vi "DangerousEnemyCriteria.vi"(8 "error in (no error)":errorcluster, 10 "Point":dbl[](array[numeric]), 11 "TestObjetive in":refnum<class "TestObjetive.lvclass">) -> (0 "error out":errorcluster, 2 "evaluation":dbl, 3 "TestObjetive out":refnum<class "TestObjetive.lvclass">)   [LabVIEW 2023, in "TestObjetive.lvclass"]
uses:
  TestObjetive.lvclass
  TestObjetive.lvclass/TestObjetive.ctl
  Game_class/Game.lvclass/Game.ctl
  Object_class/Object.lvclass/Object.ctl
  Team_class/Team.lvclass/Team.ctl
  Object_class/Read x.vi
  Object_class/Read y.vi
  Game_class/Read BallRef.vi
  Game_class/Read EnemyRef.vi
  Team_class/Read RobotRef.vi
  Object_class/Read position(x,y).vi
  Enemy_class/Enemy.lvclass
  C:/Users/ebert/Documents/codes/SSL/repo/SSL_AI/Team_class/Team.lvclass
  Ball_class/Ball.lvclass
  C:/Users/ebert/Documents/codes/SSL/repo/SSL_AI/Object_class/Object.lvclass
  Robot_class/Robot.lvclass
  Utilities_class/Utilities.lvclass
  Game_class/Game.lvclass
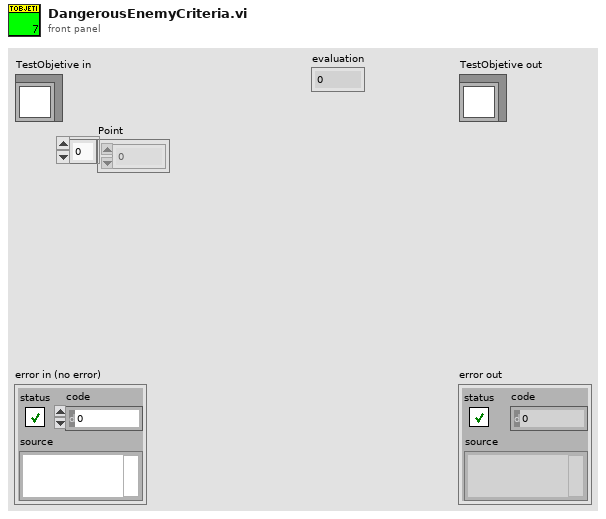
[diagram p1: front panel]
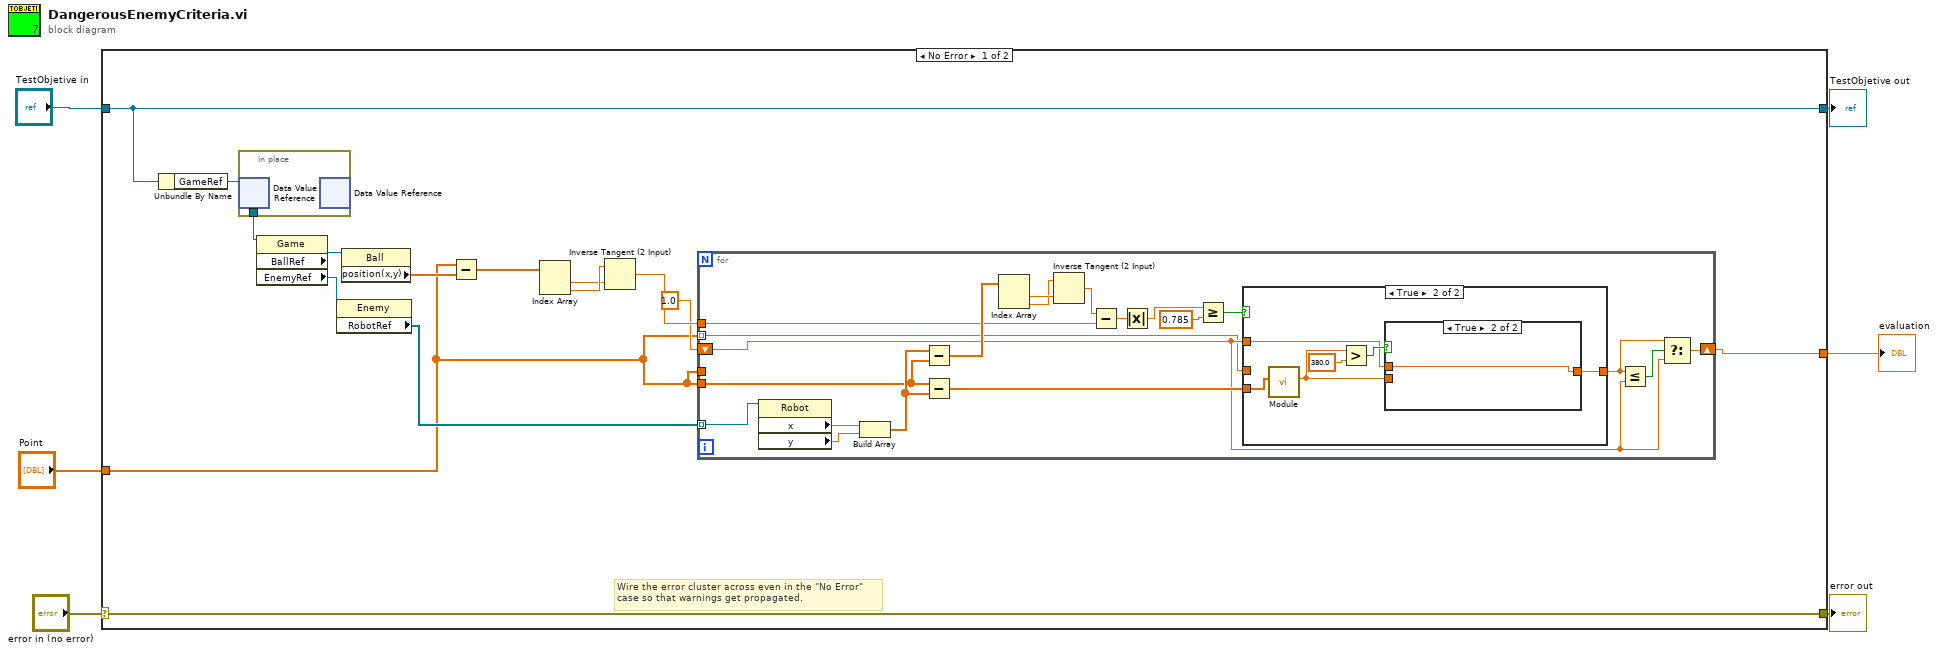
[diagram p0: block diagram]
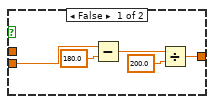
[diagram p3: hidden frame]
diagram:
  n1 = case shown="No Error" "error in (no error)" {
    selector: "error in (no error)" -> [w21 w57]
    tunnel: [w21 w57] -> w5
    tunnel: [w15 w56] -> w3
    tunnel: "TestObjetive in" -> [w15 w56]
    tunnel: "Point" -> [w8 _]
    tunnel: [w7 _] -> w1
    frame No Error {
      # "Wire the error cluster across even in the \"No Error\"\ncase so that warnings get propagated."
      n2 = Unbundle By Name(w15) -> ("GameRef"=w14:refnum<data-value>)
      n3 = in-place {
        in-place-border: [w22] -> w13
        n4 = in-place-dvr #1(w14) -> (w22:refnum<class "Game.lvclass">)  [unwired: 1 out]
        n5 = in-place-dvr #1() -> ()  [unwired: 1 in, 2 out]
      }
      n6 = property class="Game"(reference=w13) -> ("BallRef"=w12:refnum<class "Ball.lvclass">, "EnemyRef"=w10:refnum<class "Enemy.lvclass">)  [unwired: 1 in, 2 out]
      n7 = property class="Enemy"(reference=w10) -> ("RobotRef"=w9:refnum<class "Robot.lvclass">[])  [unwired: 1 in, 2 out]
      n8 = property class="Ball"(reference=w12) -> ("position(x,y)"=w11:dbl[])  [unwired: 1 in, 2 out]
      n9 = Subtract(x=w8, y=w11) -> (x-y=w20:dbl[])
      n10 = Index Array(array=w20) -> (element #1=w18:dbl, element #2=w19:dbl)  [unwired: 2 in]
      n11 = Inverse Tangent (2 Input)(1:w18, 2:w19) -> (0:w17:dbl)
      n12 = for {
        tunnel: w17 -> [w37]
        tunnel: w8 -> [_]
        shift-right: [w29] -> w7
        shift-left: 1.0 ("element") -> [w28]
        tunnel: w9 -> [w27] mode=indexing
        tunnel: w8 -> [w24] mode=indexing
        tunnel: w8 -> [w23]
        n13 = property class="Robot"(reference=w27) -> ("x"=w26:dbl, "y"=w25:dbl)  [unwired: 1 in, 2 out]
        n14 = Build Array(w26, w25) -> (w33:dbl[])
        n15 = Subtract(x=w33, y=w23) -> (x-y=w42:dbl[])
        n16 = Subtract(x=w23, y=w33) -> (x-y=w32:dbl[])
        n17 = Index Array(array=w42) -> (element #1=w39:dbl, element #2=w38:dbl)  [unwired: 2 in]
        n18 = Inverse Tangent (2 Input)(1:w39, 2:w38) -> (0:w41:dbl)
        n19 = Subtract(x=w41, y=w37) -> (x-y=w40:dbl)
        n20 = Absolute Value(x=w40) -> (abs(x)=w35:dbl)
        n21 = Greater Or Equal?(x=w35, y=0.785) -> (x >= y?=w34:bool)
        n22 = case shown="True" w34 {
          tunnel: w28 -> [w43 w46]
          tunnel: w32 -> [_ w45]
          tunnel: [w43 w48] -> w30
          tunnel: w24 -> [_ _]
          frame False {
          }
          frame True {
            n23 = call "Module.vi"("2D vector"=w45) -> ("Modulo"=w44:dbl)  [unwired: 8 in, 2 out]
            n24 = Greater?(x=w44, y=380.0) -> (0:w47:bool)
            n25 = case shown="True" w47 {
              tunnel: w46 -> [_ w55]
              tunnel: [w54 w55] -> w48
              tunnel: w44 -> [w50 _]
              frame False {
                n26 = Subtract(x=w50, y=180.0) -> (x-y=w52:dbl)
                n27 = Divide(x=w52, y=200.0) -> (x/y=w54:dbl)
              }
              frame True {
              }
            }
          }
        }
        n28 = Less Or Equal?(x=w30, y=w28) -> (x <= y?=w31:bool)
        n29 = Select(t=w30, s=w31, f=w28) -> (s? t:f=w29:dbl)
      }
    }
    frame Error {
    }
  }
  "error out" <- w5
  "TestObjetive out" <- w3
  "evaluation" <- w1
